vi "Load Effect Plugins.vi"() -> (3 "Effect Plugins":refnum<class "Effect Interface.lvclass">[](array[class]))   [LabVIEW 2019, in "Effect Unit.lvclass"]
uses:
  Effect Unit.lvclass
  Plugin Interfaces/Effect Interface/Effect Interface.lvlibp/Effect Interface Class/Effect Interface.lvclass
  <vilib>/Utility/LVLibp/NI_PackedLibraryUtility.lvlib
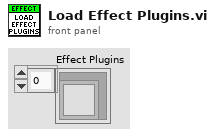
[diagram p1: front panel]
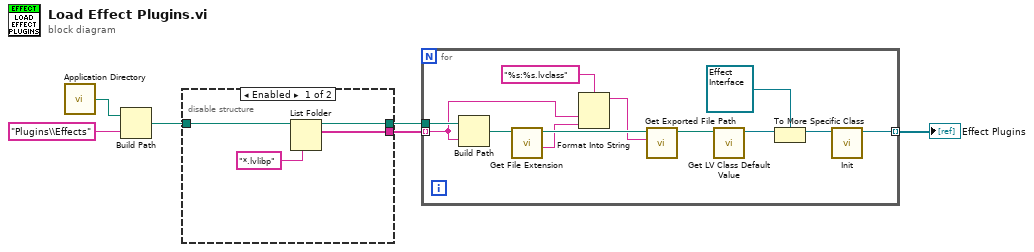
[diagram p0: block diagram]
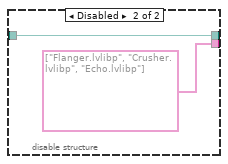
[diagram p2: hidden frame]
diagram:
  n1 = call <vilib>:"Application Directory.vi"() -> ("Application Directory"=w6:path)
  n2 = Build Path(base path=w6, name or relative path="Plugins\\Effects") -> (appended path=w4:path)
  n3 = disable-structure shown="Enabled" {
    disable-tunnel: w4 -> [w10 w11]
    disable-tunnel: [w8 string[] ["Flanger.lvlibp", "Crusher.lvlibp", "Echo.lvlibp"]] -> w3
    disable-tunnel: [w7 w11] -> w2
    frame Enabled {
      n4 = List Folder(path=w10, pattern="*.lvlibp") -> (path out=w7:path, filenames=w8:string[])  [unwired: 2 in, 2 out]
    }
    frame Disabled {
    }
  }
  n5 = for {
    tunnel: w3 -> [w19] mode=indexing
    tunnel: w2 -> [w24]
    tunnel: [w13] -> w1 mode=indexing
    n6 = Build Path(base path=w24, name or relative path=w19) -> (appended path=w23:path)
    n7 = call <vilib>:"Get File Extension.vi"("file"=w23) -> ("filename without extension"=w18:string, "dup file"=w22:path)  [unwired: 6 in, 3 out]
    n8 = Format Into String(format string="%s:%s.lvclass", w19, w18) -> (resulting string=w20:string)  [unwired: 2 in, 1 out]
    n9 = call <vilib>:"Get Exported File Path.vi"("qualified name"=w20, "packed library path"=w22) -> ("path"=w17:path)  [unwired: 8 in, 1 out]
    n10 = call <vilib>:"Get LV Class Default Value.vi"("class path"=w17) -> ("object"=w16:refnum<class>)  [unwired: 9 in, 1 out]
    n11 = To More Specific Class(target class=refnum<class "Effect Interface.lvclass"> refnum ("Effect Interface.lvlibp:Effect Interface.lvclass"), reference=w16) -> (specific class reference=w14:refnum<class "Effect Interface.lvclass">)  [unwired: 1 in, 1 out]
    n12 = call-dynamic "Init.vi"("Effect Interface in"=w14) -> ("Effect Interface out"=w13:refnum<class "Effect Interface.lvclass">)  [unwired: 9 in, 1 out]
  }
  "Effect Plugins" <- w1
